vi "T_Check.vi"(1 "Sweep\nTolerance %":dbl=0.1, 2 "T_target (K)":dbl, 3 "T_in":dbl) -> (0 "= T target":bool)   [LabVIEW 2018]
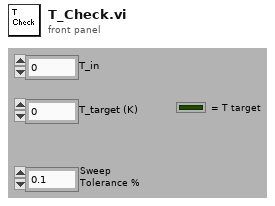
[diagram p1: front panel]
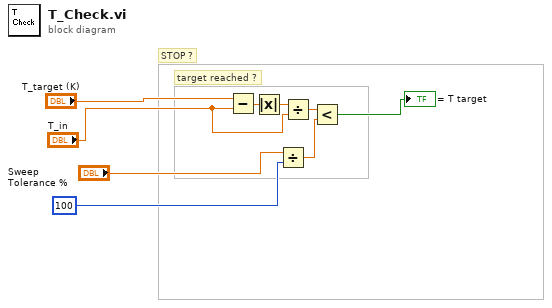
[diagram p0: block diagram]
diagram:
  # "STOP ?"
  # "target reached ?"
  n1 = Subtract(x="T_target (K)", y="T_in") -> (x-y=w9:dbl)
  n2 = Absolute Value(x=w9) -> (abs(x)=w8:dbl)
  n3 = Divide(x="Sweep\nTolerance %", y=100) -> (x/y=w6:dbl)
  n4 = Divide(x=w8, y="T_in") -> (x/y=w7:dbl)
  n5 = Less?(x=w7, y=w6) -> (x < y?=→"= T target":bool)
